vi "Array exercise.vi"() -> ()   [LabVIEW 2015]
panel:
  in  "# of Elements":i32
  in  "Start subset":i32
  in  "Scaling factor":dbl
  out "Subset Array":dbl[](array[numeric])
  out "Final Array":dbl[](array[numeric])
  out "Random Array":dbl[](array[numeric])
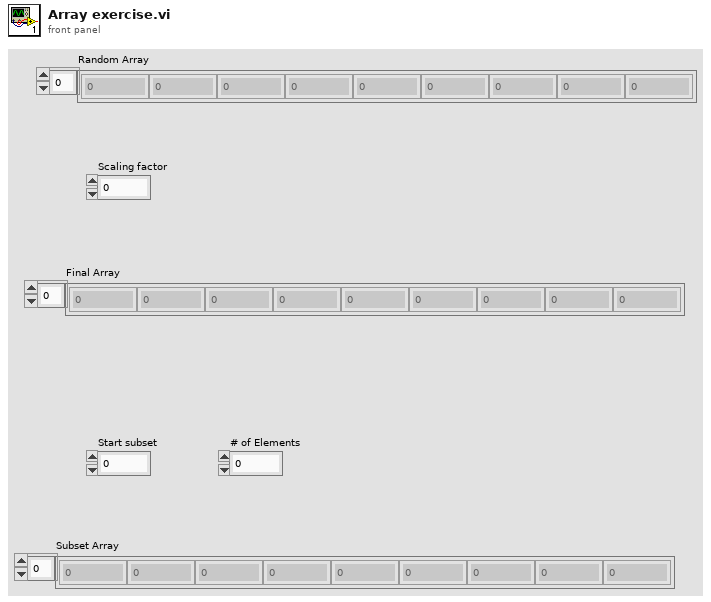
[diagram p1: front panel]
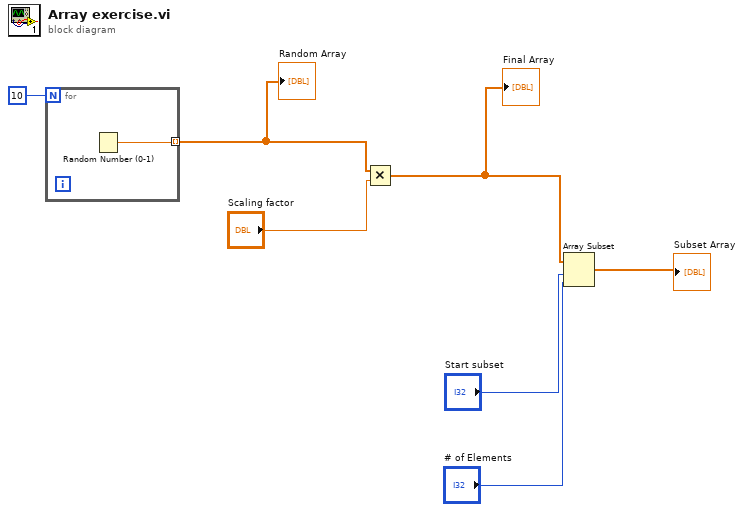
[diagram p0: block diagram]
diagram:
  n1 = for {
    N: 10 -> [_]
    tunnel: [w8] -> w6 mode=indexing
    n2 = Random Number (0-1)() -> (number: 0 to 1=w8:dbl)
  }
  "Random Array" <- w6
  n3 = Multiply(x=w6, y="Scaling factor") -> (x*y=w4:dbl[])
  "Final Array" <- w4
  n4 = Array Subset(array=w4, index="Start subset", length="# of Elements") -> (→"Subset Array":dbl[])
